vi "Application Version.vi"() -> (0 "Version":string)   [LabVIEW 2019, in "Instrument.Lockin.lvlib" / "Lockin.Utilities.lvlib"]
uses:
  Lockin.Utilities.lvlib
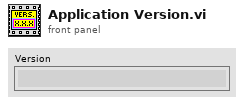
[diagram p1: front panel]
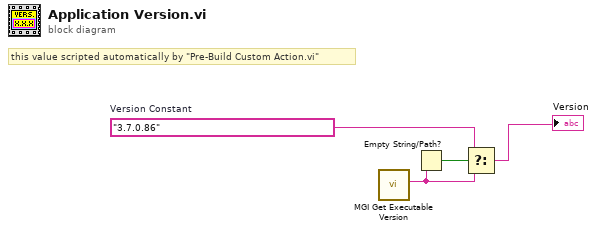
[diagram p0: block diagram]
diagram:
  w3 = "3.7.0.86"  # Version Constant
  # "this value scripted automatically by \"Pre-Build Custom Action.vi\""
  n1 = call <userlib>:"MGI Get Executable Version.vi"() -> ("Version"=w2:string)  [unwired: 7 in]
  n2 = Empty String/Path?(string/path=w2) -> (empty?=w4:bool)
  n3 = Select(t=w3, s=w4, f=w2) -> (s? t:f=→"Version":string)
